vi "SAPI_Speak_Text_File_SubVI.vi"(4 "Purge other pending text? (F)":bool, 5 "XML? (auto-detect)":T1, 6 "Wait for completion? (F)":bool, 7 "Speak Punctuation (F)":bool, 8 "error in (no error)":errorcluster, 9 "Persist any SAPI settings found in XML (F)":bool, 10 "Text file to speak":path, 11 "speech object references":T2) -> (0 "error out":errorcluster, 3 "speech object references (out)":T2)   [LabVIEW 2009]
doc: "Use the current SAPI voice settings to speak the text file wired to the 'Text file to speak' input."
uses:
  Controls/Speech object references.ctl
  Controls/SAPI_Speak_Method_XML_Flag_Enum.ctl
  SAPI.TTS.lvlib
panel:
  # "Use the current SAPI voice settings to speak\nthe text string wired to the Text input."
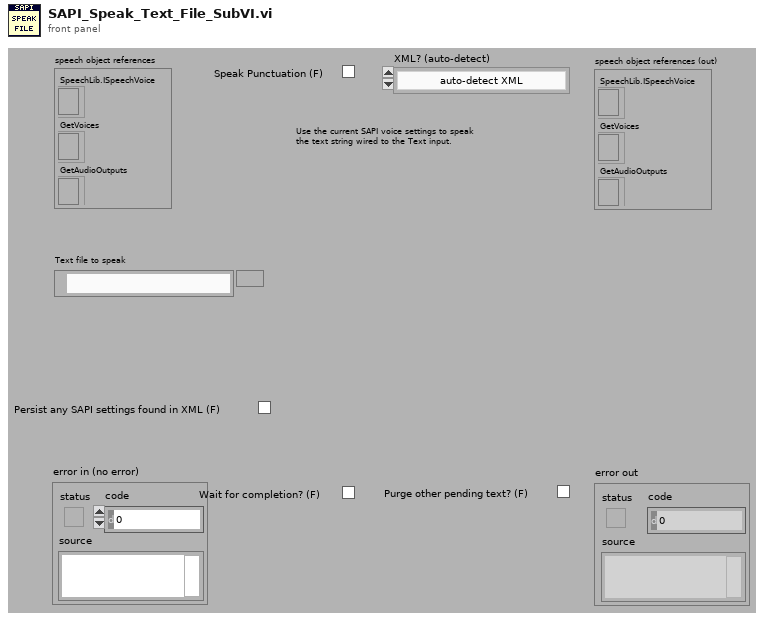
[diagram p1: front panel]
types:
  T1 = typedef "SAPI_Speak_Method_XML_Flag_Enum.ctl" = enum16{"auto-detect XML", "always treat input as XML", "never treat input as XML"}
  T2 = typedef "SAPI.TTS.lvlib/Speech object references.ctl" = cluster{"SpeechLib.ISpeechVoice":refnum<k7>, "GetVoices":refnum<k7>, "GetAudioOutputs":refnum<k7>}
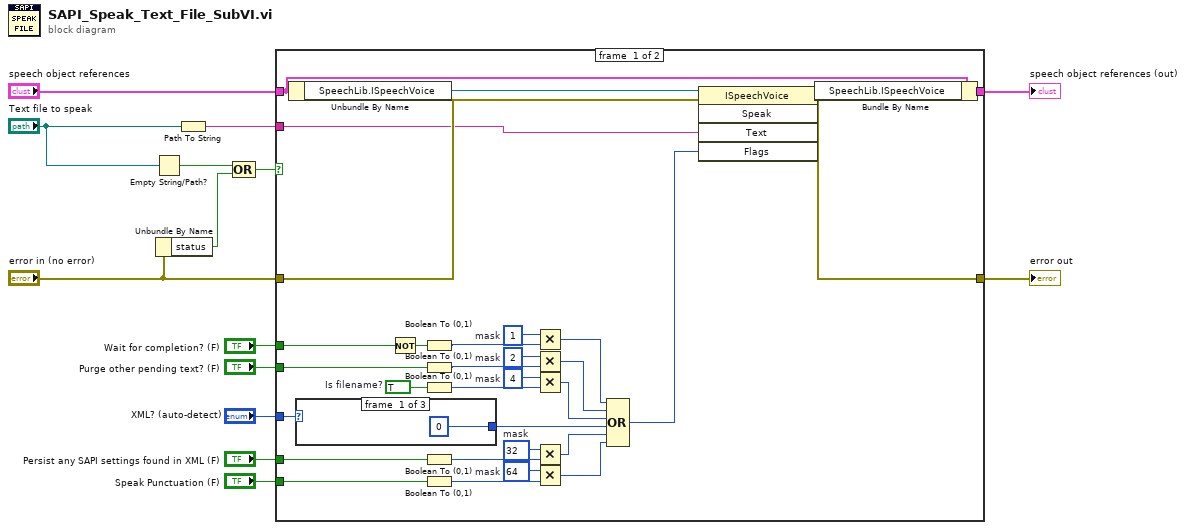
[diagram p0: block diagram]
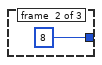
[diagram p2: hidden frame]
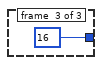
[diagram p3: hidden frame]
diagram:
  n1 = Empty String/Path?(string/path="Text file to speak") -> (empty?=w10:bool)
  n2 = Unbundle By Name("error in (no error)") -> ("status"=w9:bool)
  n3 = Path To String(path="Text file to speak") -> (string=w2:string)
  n4 = Compound Arithmetic op=OR(w10, w9) -> (w3:bool)
  n5 = case shown="False" w3 {
    tunnel: "speech object references" -> [w45 w49]
    tunnel: [w44 w50] -> w13
    tunnel: [w43 w49] -> w12
    tunnel: "error in (no error)" -> [w42 w50]
    tunnel: "Wait for completion? (F)" -> [w40 _]
    tunnel: "Speak Punctuation (F)" -> [w38 _]
    tunnel: "Persist any SAPI settings found in XML (F)" -> [w37 _]
    tunnel: "Purge other pending text? (F)" -> [w36 _]
    tunnel: "XML? (auto-detect)" -> [w21 _]
    tunnel: w2 -> [w18 _]
    frame #0 {
      w15 = TRUE  # Is filename?
      w31 = 64  # mask
      w32 = 32  # mask
      w33 = 4  # mask
      w34 = 2  # mask
      w41 = 1  # mask
      n6 = Unbundle By Name(w45) -> ("SpeechLib.ISpeechVoice"=w17:refnum<k7>)
      n7 = case shown="\"auto-detect XML\"" w21 {
        tunnel: [0 8 16] -> w20
        frame #0 {
        }
        frame #1 {
        }
        frame #2 {
        }
      }
      n8 = Not(x=w40) -> (.not. x?=w39:bool)
      n9 = Boolean To (0,1)(Boolean=w39) -> (0, 1=w35:i16)
      n10 = Boolean To (0,1)(Boolean=w36) -> (0, 1=w27:i16)
      n11 = Boolean To (0,1)(Boolean=w15) -> (0, 1=w28:i16)
      n12 = Boolean To (0,1)(Boolean=w37) -> (0, 1=w29:i16)
      n13 = Boolean To (0,1)(Boolean=w38) -> (0, 1=w30:i16)
      n14 = Multiply(x=w41, y=w35) -> (x*y=w26:i32)
      n15 = Multiply(x=w34, y=w27) -> (x*y=w25:i32)
      n16 = Multiply(x=w33, y=w28) -> (x*y=w24:i32)
      n17 = Multiply(x=w32, y=w29) -> (x*y=w23:i32)
      n18 = Multiply(x=w31, y=w30) -> (x*y=w19:i32)
      n19 = Compound Arithmetic op=OR(w26, w25, w24, w20, w23, w19) -> (w22:i32)
      n20 = invoke class="ISpeechVoice" method="Speak"(reference=w17, error in=w42, "Text"=w18, "Flags"=w22) -> (reference out=w16:refnum<k7>, error out=w44:errorcluster)  [unwired: 1 in, 3 out]
      n21 = Bundle By Name(cluster=w45, "SpeechLib.ISpeechVoice"=w16) -> (w43:T2)
    }
    frame #1 {
    }
  }
  "error out" <- w13
  "speech object references (out)" <- w12
